vi "Legend Palette.vi"(4 "Active Plot":i32, 6 "Control Ref Queue":T4, 9 "Window Bounds":T5, 10 "Multiplot Representation In":T1, 11 "2D Compass.lvclass in":refnum<class "2D Compass.lvclass">) -> (1 "Cancel?":bool, 2 "Multiplot Representation Out":T1, 3 "2D Compass.lvclass out":refnum<class "2D Compass.lvclass">)   [LabVIEW 2020, in "2D Compass.lvclass"]
uses:
  <vilib>/Math Plots/2D Math Plots/2D Compass/2D Compass/2D Compass.lvclass
  e:/builds/penguin/labview/branches/2020/dev/dist/vi.lib/Math Plots/2D Math Plots/2D Plot/2D Plot/2D Plot.lvclass
  <vilib>/Math Plots/2D Math Plots/2D Plot/Action String/2DMathPlot Ctrl Act Queue.ctl
  <vilib>/Math Plots/2D Math Plots/2D Plot/Action String/2DMathPlot Ctrl Act Cluster.ctl
  <vilib>/Math Plots/2D Math Plots/2D Plot/Action String/2DMathPlot State Class.ctl
  <vilib>/Math Plots/2D Math Plots/2D Plot/2D Plot/Typedef/Multiplot Representation.ctl
  <vilib>/Math Plots/2D Math Plots/2D Plot/2D Plot/Typedef/Plot Representation.ctl
  <vilib>/Math Plots/2D Math Plots/2D Plot/2D Plot/Typedef/Range Cluster.ctl
  <vilib>/Utility/miscctls.llb/LVRectTypeDef.ctl
  <vilib>/Math Plots/2D Math Plots/2D Compass/2D Compass/2D Compass.lvclass/2D Compass.ctl
  <vilib>/Math Plots/2D Math Plots/2D Plot/2D Plot/2D Plot.lvclass
panel:
  in  "Tab Control":enum32{"Plot Property", "Input & Output"}(tab)
  in  "Line Width":u16(ring) caption="Line width"
  in  "Line Style":u16(ring) caption="Line style"
  in  "OK":bool
  in  "Cancel":bool
  in  "Compass size":dbl
  in  "Compass Color":u32(colorbox)
  # "Line style"
  # "Line width"
  # "Compass size"
  # "Compass color"
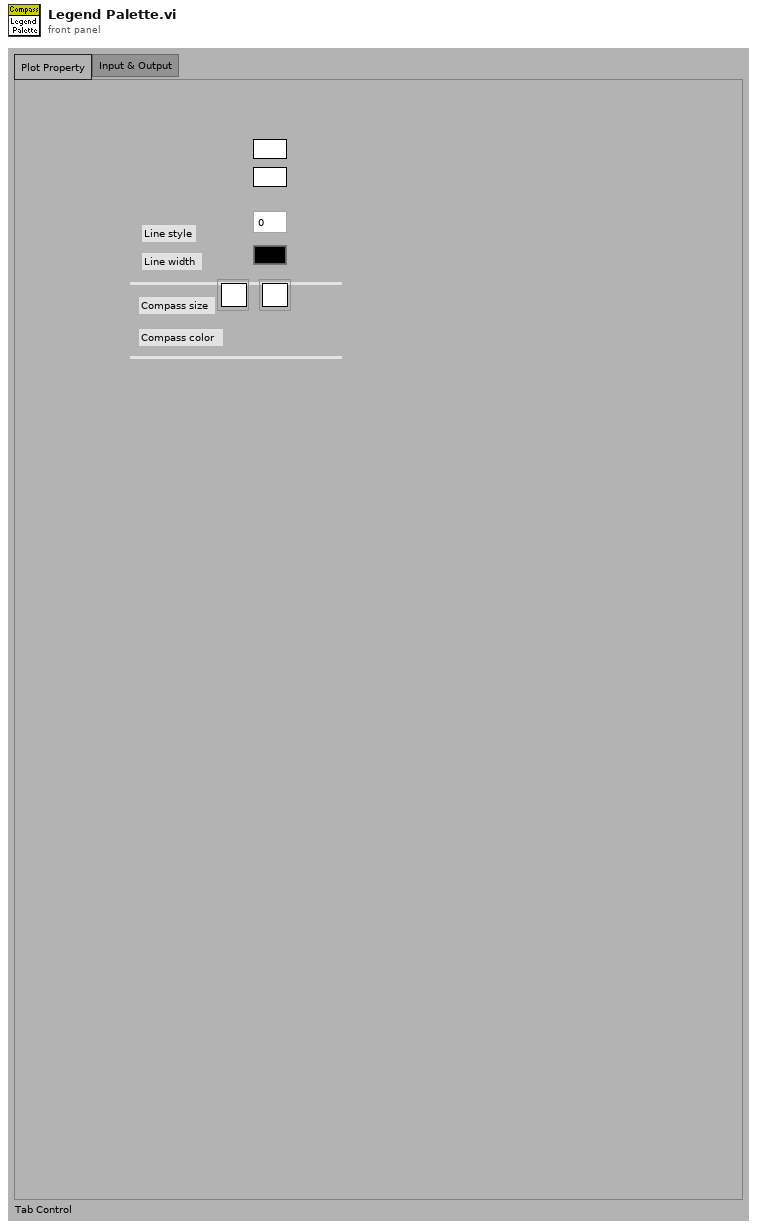
[diagram p1: front panel]
types:
  T1 = typedef "2D Plot.lvclass/Multiplot Representation.ctl" = cluster{"Plot Representation Array":T2[], "Max Range":T3}
  T2 = typedef "2D Plot.lvclass/Plot Representation.ctl" = cluster{"Plot Range":T3, "Vertex Cluster":cluster{"Vertex X Array":dbl[], "Vertex Y Array":dbl[]}, "Base Cluster":cluster{"Base X Array":dbl[], "Base Y Array":dbl[]}}
  T3 = typedef "2D Plot.lvclass/Range Cluster.ctl" = cluster{"X Range":cluster{"Max X":dbl, "Min X":dbl}, "Y Range":cluster{"Max Y":dbl, "Min Y":dbl}}
  T4 = typedef "2DMathPlot Ctrl Act Queue.ctl" = refnum<queue>
  T5 = typedef "LVRectTypeDef.ctl" = cluster{"Left":i16, "Top":i16, "Right":i16, "Bottom":i16}
  T6 = typedef "2DMathPlot Ctrl Act Cluster.ctl" = cluster{"Plot Area Ref":refnum<vi>, "Z Axis Ref":refnum<vi>, "Legend Ref":refnum<vi>, "XControl Ref":refnum<vi>, "Facade Ref":refnum<vi>, "Display State Change Class":T7}
  T7 = typedef "2DMathPlot State Class.ctl" = enum16{"Update All (Undo)", "Update General", "Update Appearance", "Update Format", "Update Scale", "Update Marker", "Update Cursor", "None"}
  T8 = typedef "2D Plot.lvclass/Plot Property Array.ctl" = T9[]
  T9 = typedef "2D Plot.lvclass/Plot Property.ctl" = cluster{"Bar Plot Style":u8, "DigitalLineStyle":u8, "TransitionLocation":u8, "Transition Type":u8, "Fill To":i16, "Fill/Pt. Color":u32, "Label Style":u8, "Line Style":u8, "Line Width":u8, "Plot Color":u32, "Plot Interpolation":u8, "Plot Name":string, "Point Style":u8, "Visible?":bool, "XScaleIdx":u32, "YScaleIdx":u32}
  T10 = typedef "2D Compass.lvclass/2D Compass Property Array.ctl" = T11[]
  T11 = typedef "2D Compass.lvclass/2D Compass Property.ctl" = cluster{"Compass Size":dbl}
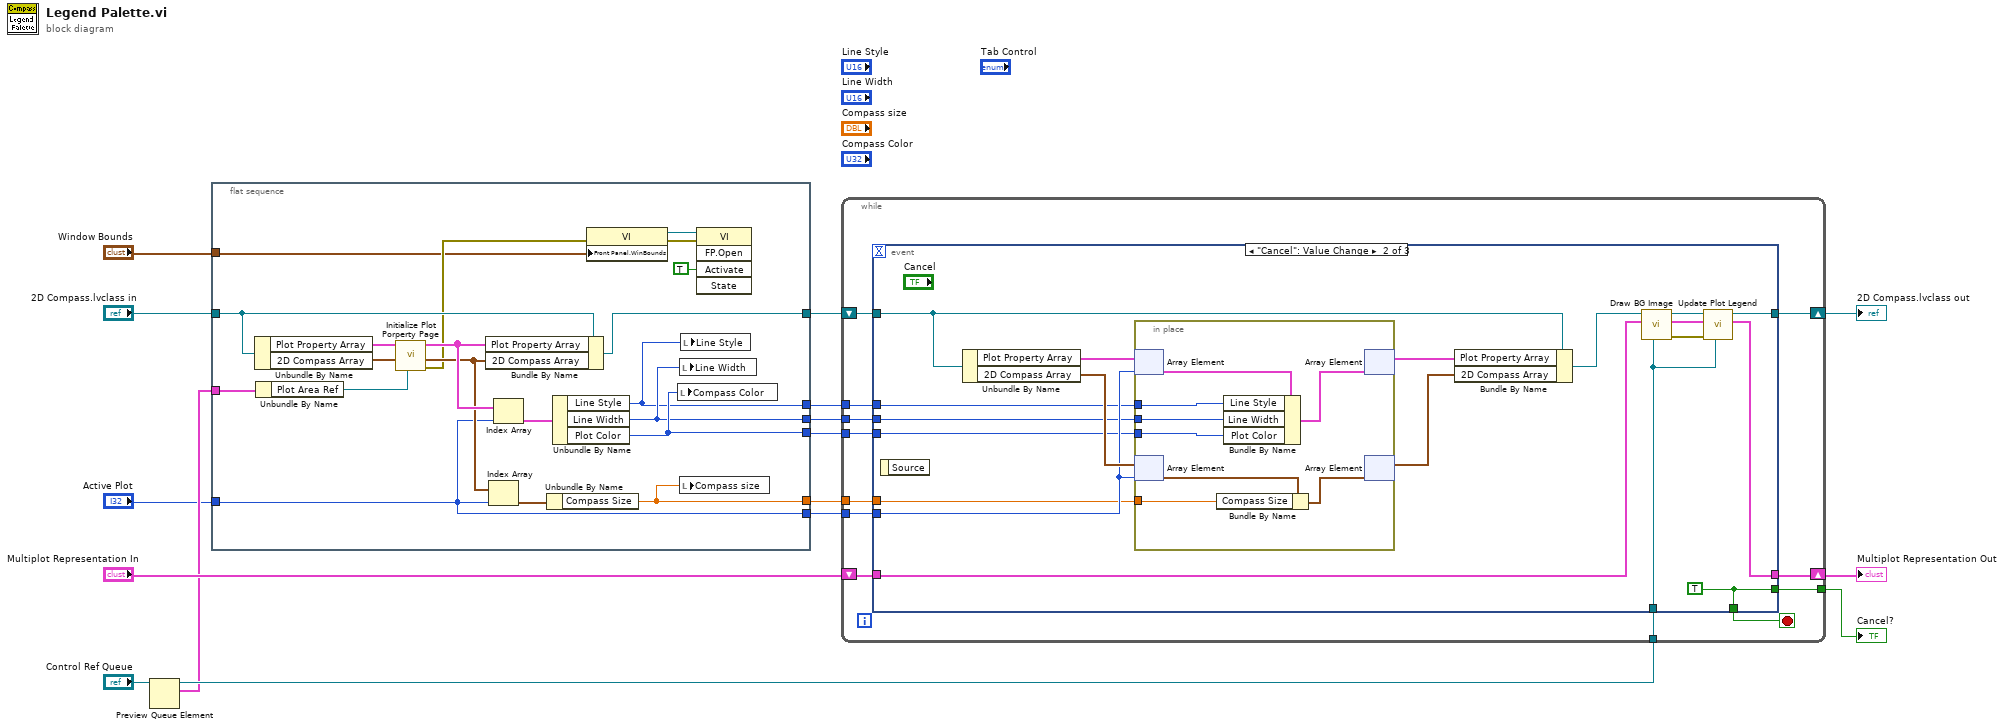
[diagram p0: block diagram]
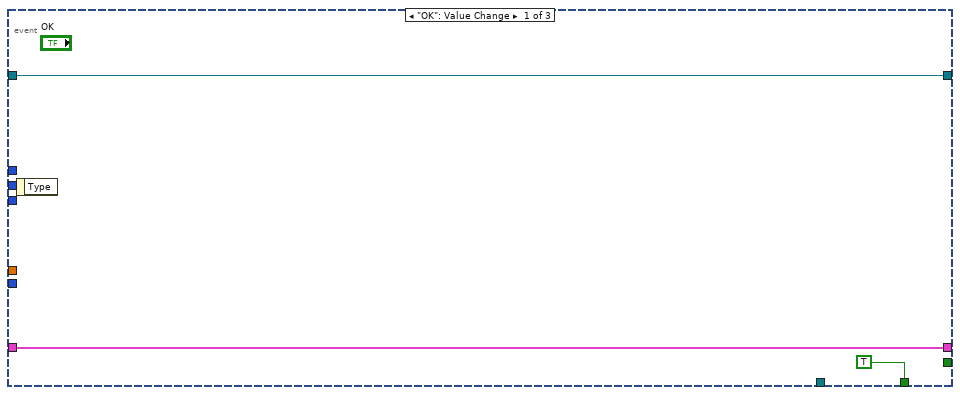
[diagram p2: hidden frame]
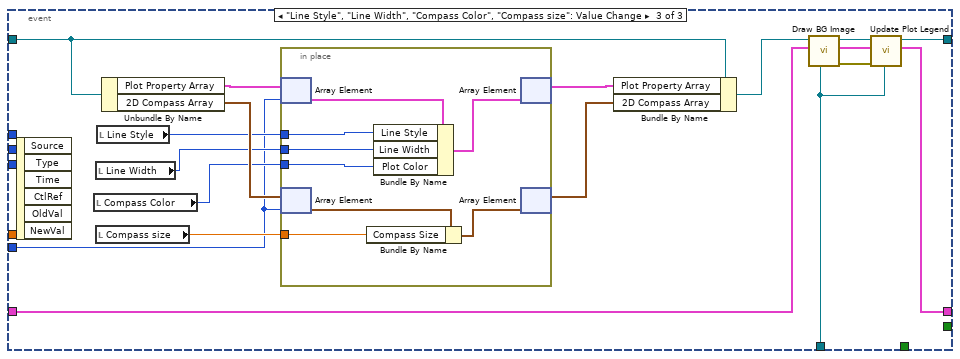
[diagram p3: hidden frame]
diagram:
  n1 = Preview Queue Element(queue="Control Ref Queue") -> (queue out=w10:T4, element=w9:T6)  [unwired: 1 in, 3 out]
  n2 = flat-sequence {
    tunnel: "2D Compass.lvclass in" -> [w24]
    tunnel: [w23] -> w14
    tunnel: [w20] -> w4
    tunnel: w9 -> [w34]
    tunnel: [w33] -> w8
    tunnel: [w32] -> w7
    tunnel: [w31] -> w6
    tunnel: [w30] -> w5
    tunnel: "Window Bounds" -> [w21]
    tunnel: "Active Plot" -> [w20]
    frame #0 {
      n3 = Unbundle By Name(w24) -> ("Plot Property Array"=w29:T8, "2D Compass Array"=w28:T10)
      n4 = Unbundle By Name(w34) -> ("Plot Area Ref"=w27:refnum<vi>)
      n5 = call <vilib>:"Initialize Plot Porperty Page.vi"("Plot Area Ref"=w27, "2D Compass Array In"=w28, "Plot Property Array In"=w29) -> ("error out"=w22:errorcluster, "2D Compass Array Out"=w25:T10, "Plot Property Array Out"=w26:T8)  [unwired: 2 in, 4 out]
      n6 = Bundle By Name(cluster=w24, "Plot Property Array"=w26, "2D Compass Array"=w25) -> (w23:refnum<class "2D Compass.lvclass">)
      n7 = Index Array(array=w25, index=w20) -> (element=w35:T11)
      n8 = Index Array(array=w26, index=w20) -> (element=w36:T9)
      n9 = Unbundle By Name(w35) -> ("Compass Size"=w33:dbl)
      n10 = Unbundle By Name(w36) -> ("Line Style"=w30:u8, "Line Width"=w31:u8, "Plot Color"=w32:u32)
      n11 = property class="VI"(error in=w22, "Front Panel.WinBounds"=w21) -> (reference out=w18:refnum<vi>, error out=w19:errorcluster)  [unwired: 1 in]
      n12 = local write "Compass Color"(w32) -> ()
      n13 = local write "Line Width"(w31) -> ()
      n14 = local write "Compass size"(w33) -> ()
      n15 = local write "Line Style"(w30) -> ()
      n16 = invoke class="VI" method="FP.Open"(reference=w18, error in=w19, "Activate"=TRUE ("Activate?")) -> ()  [unwired: 2 in, 5 out]
    }
  }
  n17 = while {
    shift-right: [w47] -> w16
    shift-left: w14 -> [w48]
    shift-right: [w45] -> w12
    shift-left: "Multiplot Representation In" -> [w46]
    tunnel: w10 -> [w44]
    tunnel: w4 -> [w43]
    tunnel: w8 -> [w41]
    tunnel: w7 -> [w40]
    tunnel: w6 -> [w39]
    tunnel: w5 -> [w38]
    tunnel: [w37] -> w3
    stop <- w42 stop-if-true
    n18 = event shown="[1] \"Cancel\": Value Change" {
      selector: _ -> [_ _ _]
      dyn-events: _ -> [_ _ _]
      timeout: _ -> [_ _ _]
      tunnel: w48 -> [w51 w65 w94]
      tunnel: [w51 w55 w83] -> w47
      tunnel: w46 -> [w50 w64 w86]
      tunnel: [w50 w53 w81] -> w45
      tunnel: w44 -> [_ w54 w80]
      tunnel: w43 -> [_ w63 w85]
      tunnel: [TRUE w52 _] -> w42
      tunnel: w41 -> [_ w62 _]
      tunnel: w40 -> [_ w61 _]
      tunnel: w39 -> [_ w60 _]
      tunnel: w38 -> [_ w59 _]
      tunnel: [_ w52 _] -> w37
      event "OK": Value Change {
        n19 = event-data() -> ()  [unwired: 2 out]
      }
      event "Cancel": Value Change {
        w52 = TRUE
        n20 = event-data() -> ()  [unwired: 2 out]
        n21 = Unbundle By Name(w65) -> ("Plot Property Array"=w70:T8, "2D Compass Array"=w69:T10)
        n22 = in-place {
          in-place-border: w62 -> [w74]
          in-place-border: w59 -> [w73]
          in-place-border: w60 -> [w72]
          in-place-border: w61 -> [w71]
          n23 = in-place-array #1(w70, w63) -> (w78:T9)
          n24 = in-place-array #2(w69, w63) -> (w77:T11)
          n25 = Bundle By Name(cluster=w77, "Compass Size"=w74) -> (w76:T11)
          n26 = Bundle By Name(cluster=w78, "Line Style"=w73, "Line Width"=w72, "Plot Color"=w71) -> (w75:T9)
          n27 = in-place-array #1(w75) -> (w68:T8)  [unwired: 1 out]
          n28 = in-place-array #2(w76) -> (w67:T10)  [unwired: 1 out]
        }
        n29 = Bundle By Name(cluster=w65, "Plot Property Array"=w68, "2D Compass Array"=w67) -> (w66:refnum<class "2D Compass.lvclass">)
        n30 = call-dynamic "Draw BG Image.vi"("Control Ref Queue"=w54, "Multiplot Representation In"=w64, "2D Compass.lvclass in"=w66) -> ("error out"=w56:errorcluster, "Multiplot Representation Out"=w57:T1, "2D Compass.lvclass out"=w58:refnum<class "2D Compass.lvclass">)  [unwired: 1 in, 5 out]
        n31 = call <vilib>:"Update Plot Legend.vi"("Control Ref Queue"=w54, "error in (no error)"=w56, "Multiplot Representation In"=w57, "2D Plot in"=w58) -> ("Multiplot Representation Out"=w53:T1, "2D Plot out"=w55:refnum<class "2D Compass.lvclass">)  [unwired: 6 out]
      }
      event "Line Style", "Line Width", "Compass Color", "Compass size": Value Change {
        n32 = event-data() -> ()  [unwired: 7 out]
        n33 = local read "Compass Color"() -> (w88:u32)
        n34 = local read "Line Width"() -> (w89:u16)
        n35 = local read "Compass size"() -> (w91:dbl)
        n36 = local read "Line Style"() -> (w90:u16)
        n37 = Unbundle By Name(w94) -> ("Plot Property Array"=w96:T8, "2D Compass Array"=w95:T10)
        n38 = in-place {
          in-place-border: w91 -> [w100]
          in-place-border: w90 -> [w99]
          in-place-border: w89 -> [w98]
          in-place-border: w88 -> [w97]
          n39 = in-place-array #3(w96, w85) -> (w104:T9)
          n40 = in-place-array #4(w95, w85) -> (w103:T11)
          n41 = Bundle By Name(cluster=w103, "Compass Size"=w100) -> (w102:T11)
          n42 = Bundle By Name(cluster=w104, "Line Style"=w99, "Line Width"=w98, "Plot Color"=w97) -> (w101:T9)
          n43 = in-place-array #3(w101) -> (w93:T8)  [unwired: 1 out]
          n44 = in-place-array #4(w102) -> (w92:T10)  [unwired: 1 out]
        }
        n45 = Bundle By Name(cluster=w94, "Plot Property Array"=w93, "2D Compass Array"=w92) -> (w87:refnum<class "2D Compass.lvclass">)
        n46 = call-dynamic "Draw BG Image.vi"("Control Ref Queue"=w80, "Multiplot Representation In"=w86, "2D Compass.lvclass in"=w87) -> ("error out"=w79:errorcluster, "Multiplot Representation Out"=w82:T1, "2D Compass.lvclass out"=w84:refnum<class "2D Compass.lvclass">)  [unwired: 1 in, 5 out]
        n47 = call <vilib>:"Update Plot Legend.vi"("Control Ref Queue"=w80, "error in (no error)"=w79, "Multiplot Representation In"=w82, "2D Plot in"=w84) -> ("Multiplot Representation Out"=w81:T1, "2D Plot out"=w83:refnum<class "2D Compass.lvclass">)  [unwired: 6 out]
      }
    }
  }
  "2D Compass.lvclass out" <- w16
  "Multiplot Representation Out" <- w12
  "Cancel?" <- w3
